vi "Initial Values-format and values-Live window.vi"() -> (13 "Values.Boolean":bool[](array[boolean]), 14 "Keys setup.DBL":T2=[{"key"="Control FPGA.Clock Freq (MHz)", "Save?"=TRUE, "Default"=240.0}, {"key"="DAQ FPGA.Clock Freq (MHz)", "Save?"=TRUE, "Default"=240.0}], 15 "Values.DBL":dbl[](array[numeric]), 16 "Keys setup.String":T3=[{"key"="Control FPGA.MAC address", "Save?"=TRUE, "Default"="AABBCCDDEEFF"}, {"key"="DAQ FPGA.Target", "Save?"=TRUE, "Default"="RIO0"}, {"key"="XY Stage.COM port", "Save?"=TRUE, "Default"="COM7"}, {"key"="DAQmx Chan.Pockels Control", "Save?"=TRUE, "Default"=""}, {"key"="DAQmx Chan.Hard Shutter", "Save?"=TRUE, "Default"=""}, {"key"="DAQmx Chan.PMT 1", "Save?"=TRUE, "Default"=""}, {"key"="DAQmx Chan.PMT 2", "Save?"=TRUE, "Default"=""}, {"key"="DAQmx Chan.Encoder Trigger", "Save?"=TRUE, "Default"=""}, {"key"="DAQmx Chan.Optional Trigger 1", "Save?"=TRUE, "Default"=""}, {"key"="DAQmx Chan.Optional Trigger 2", "Save?"=TRUE, "Default"=""}, {"key"="DAQmx Chan.Optional Trigger 3", "Save?"=TRUE, "Default"=""}], 17 "Values.Strings":string[](array[string]), 18 "Keys setup.Boolean":T1, 19 "error out":errorcluster)   [LabVIEW 2017]
uses:
  Typedefs/Ini file interface (String).ctl
  Typedefs/Ini file interface (DBL).ctl
  Typedefs/Ini file interface (Boolean).ctl
  User Interface/Globals/gl_Windows Ctrl refs.vi
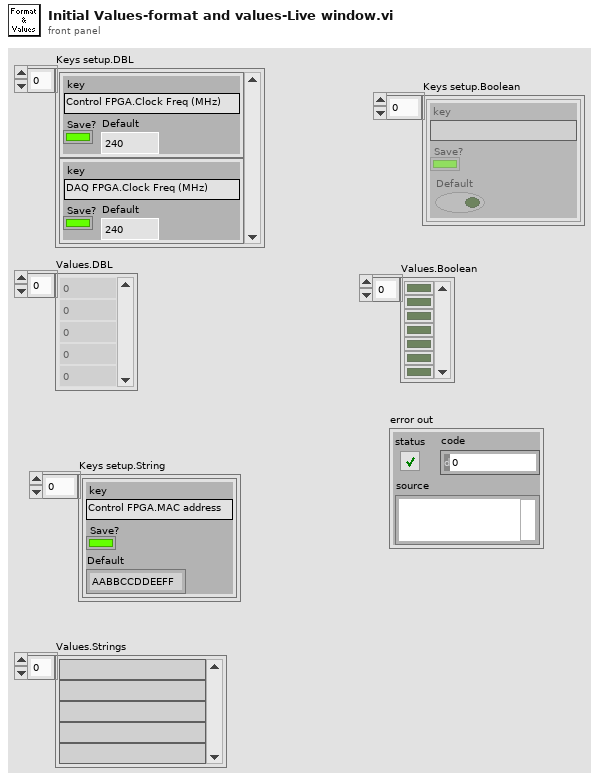
[diagram p1: front panel]
types:
  T1 = typedef "Ini file interface (Boolean).ctl" = cluster{"key":string, "Save?":bool, "Default":bool}[]
  T2 = typedef "Ini file interface (DBL).ctl" = cluster{"key":string, "Save?":bool, "Default":dbl}[]
  T3 = typedef "Ini file interface (String).ctl" = cluster{"key":string, "Save?":bool, "Default":string}[]
  T4 = typedef "Live window-ctrl refs.ctl" = cluster{"This VI":refnum<vi>, "Pane":refnum<vi>, "Show REF Image Left":refnum<vi>, "Show REF Image Right":refnum<vi>, "Snapshot":refnum<vi>, "Left Image Palette":refnum<vi>, "Right Image Palette":refnum<vi>, "Left Channel":refnum<vi>, "Right Channel":refnum<vi>, "Left image intensity":refnum<vi>, "Right image intensity":refnum<vi>, "Left Image Display":T5, "Right Image Display":T5, "Refresh rate ind (Hz)":refnum<vi>, "Acq rate ind (Hz)":refnum<vi>, "Stop (ind)":refnum<vi>}
  T5 = typedef "Image display ref.ctl" = refnum<vi>
  T6 = typedef "Channel Selector.ctl" = enum16{"Red Channel", "Green Channel", "Blended"}
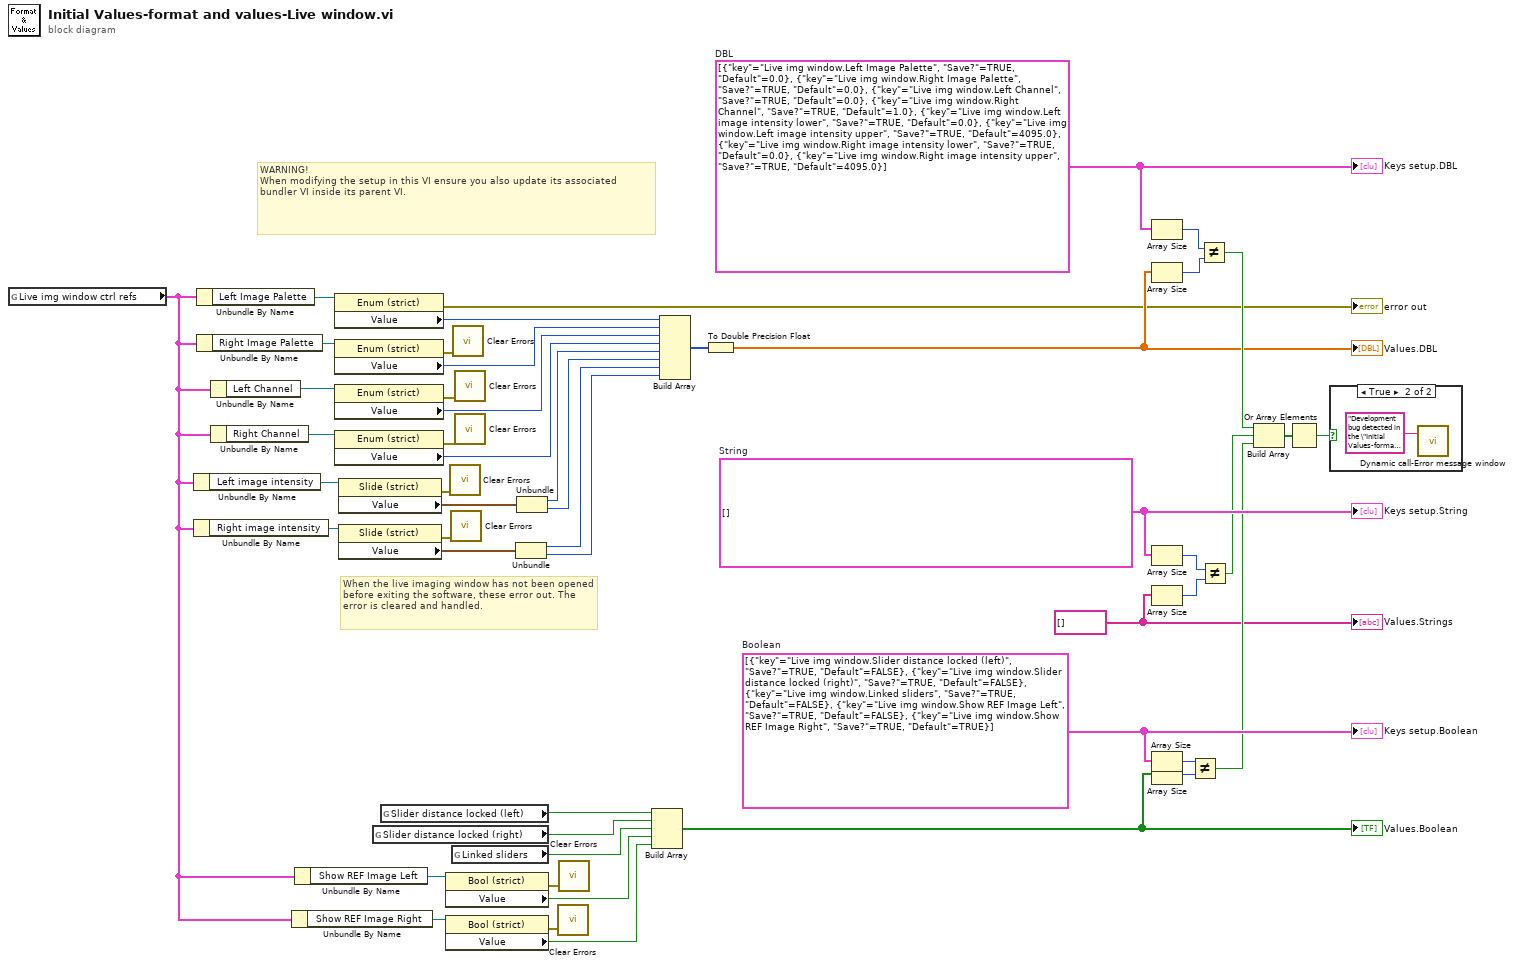
[diagram p0: block diagram]
diagram:
  w34 = string[] [] ("appended array")
  w47 = T1 [{"key"="Live img window.Slider distance locked (left)", "Save?"=TRUE, "Default"=FALSE}, {"key"="Live img window.Slider distance locked (right)", "Save?"=TRUE, "Default"=FALSE}, {"key"="Live img window.Linked sliders", "Save?"=TRUE, "Default"=FALSE}, {"key"="Live img window.Show REF Image Left", "Save?"=TRUE, "Default"=FALSE}, {"key"="Live img window.Show REF Image Right", "Save?"=TRUE, "Default"=TRUE}]  # Boolean
  w50 = T3 []  # String
  w49 = T2 [{"key"="Live img window.Left Image Palette", "Save?"=TRUE, "Default"=0.0}, {"key"="Live img window.Right Image Palette", "Save?"=TRUE, "Default"=0.0}, {"key"="Live img window.Left Channel", "Save?"=TRUE, "Default"=0.0}, {"key"="Live img window.Right Channel", "Save?"=TRUE, "Default"=1.0}, {"key"="Live img window.Left image intensity lower", "Save?"=TRUE, "Default"=0.0}, {"key"="Live img window.Left image intensity upper", "Save?"=TRUE, "Default"=4095.0}, {"key"="Live img window.Right image intensity lower", "Save?"=TRUE, "Default"=0.0}, {"key"="Live img window.Right image intensity upper", "Save?"=TRUE, "Default"=4095.0}]  # DBL
  # "When the live imaging window has not been opened before exiting the software, these error out. The error is cleared and handled."
  # "WARNING!\nWhen modifying the setup in this VI ensure you also update its associated bundler VI inside its parent VI."
  n1 = global read "gl_Windows Ctrl refs.vi" "Live img window ctrl refs"() -> (w5:T4)
  n2 = Unbundle By Name(w5) -> ("Left image intensity"=w24:refnum<vi>)
  n3 = Unbundle By Name(w5) -> ("Right image intensity"=w25:refnum<vi>)
  n4 = Unbundle By Name(w5) -> ("Left Image Palette"=w35:refnum<vi>)
  n5 = Unbundle By Name(w5) -> ("Right Image Palette"=w32:refnum<vi>)
  n6 = Unbundle By Name(w5) -> ("Left Channel"=w29:refnum<vi>)
  n7 = Unbundle By Name(w5) -> ("Right Channel"=w30:refnum<vi>)
  n8 = Unbundle By Name(w5) -> ("Show REF Image Right"=w6:refnum<vi>)
  n9 = Unbundle By Name(w5) -> ("Show REF Image Left"=w7:refnum<vi>)
  n10 = property class="Enum (strict)"(reference=w35) -> (error out=→"error out":errorcluster, "Value"=w33:enum16{"Gray", "Red", "Green"})  [unwired: 1 in, 1 out]
  n11 = property class="Enum (strict)"(reference=w32) -> (error out=w17:errorcluster, "Value"=w31:enum16{"Gray", "Red", "Green"})  [unwired: 1 in, 1 out]
  n12 = property class="Enum (strict)"(reference=w29) -> (error out=w16:errorcluster, "Value"=w28:T6)  [unwired: 1 in, 1 out]
  n13 = property class="Enum (strict)"(reference=w30) -> (error out=w15:errorcluster, "Value"=w27:T6)  [unwired: 1 in, 1 out]
  n14 = property class="Slide (strict)"(reference=w24) -> (error out=w14:errorcluster, "Value"=w23:cluster{i16, i16})  [unwired: 1 in, 1 out]
  n15 = property class="Slide (strict)"(reference=w25) -> (error out=w13:errorcluster, "Value"=w22:cluster{i16, i16})  [unwired: 1 in, 1 out]
  n16 = global read "gl_Windows Ctrl refs.vi" "Slider distance locked (right)"() -> (w10:bool)
  n17 = global read "gl_Windows Ctrl refs.vi" "Slider distance locked (left)"() -> (w11:bool)
  n18 = property class="Bool (strict)"(reference=w7) -> (error out=w2:errorcluster, "Value"=w4:bool)  [unwired: 1 in, 1 out]
  n19 = property class="Bool (strict)"(reference=w6) -> (error out=w1:errorcluster, "Value"=w3:bool)  [unwired: 1 in, 1 out]
  n20 = call <vilib>:"Clear Errors.vi"("error in (no error)"=w14) -> ()  [unwired: 5 in, 2 out]
  n21 = call <vilib>:"Clear Errors.vi"("error in (no error)"=w13) -> ()  [unwired: 5 in, 2 out]
  n22 = global read "gl_Windows Ctrl refs.vi" "Linked sliders"() -> (w8:bool)
  n23 = call <vilib>:"Clear Errors.vi"("error in (no error)"=w17) -> ()  [unwired: 5 in, 2 out]
  n24 = call <vilib>:"Clear Errors.vi"("error in (no error)"=w16) -> ()  [unwired: 5 in, 2 out]
  n25 = call <vilib>:"Clear Errors.vi"("error in (no error)"=w15) -> ()  [unwired: 5 in, 2 out]
  n26 = Unbundle(w22) -> (w19:i16, w18:i16)
  n27 = Unbundle(w23) -> (w21:i16, w20:i16)
  n28 = call <vilib>:"Clear Errors.vi"("error in (no error)"=w1) -> ()  [unwired: 5 in, 2 out]
  n29 = call <vilib>:"Clear Errors.vi"("error in (no error)"=w2) -> ()  [unwired: 5 in, 2 out]
  n30 = Build Array(w11, w10, w8, w4, w3) -> (w9:bool[])
  "Values.Boolean" <- w9
  n31 = Build Array(w33, w31, w28, w27, w21, w20, w19, w18) -> (w48:u16[])
  n32 = To Double Precision Float(number=w48) -> (double precision float=w26:dbl[])
  "Values.DBL" <- w26
  n33 = Array Size(array=w49) -> (size(s)=w44:i32)
  n34 = Array Size(array=w26) -> (size(s)=w43:i32)
  n35 = Array Size(array=w50) -> (size(s)=w46:i32)
  n36 = Array Size(array=w34) -> (size(s)=w45:i32)
  n37 = Array Size(array=w47) -> (size(s)=w42:i32)
  n38 = Array Size(array=w9) -> (size(s)=w41:i32)
  n39 = Not Equal?(x=w42, y=w41) -> (x != y?=w39:bool)
  n40 = Not Equal?(x=w44, y=w43) -> (x != y?=w37:bool)
  n41 = Not Equal?(x=w46, y=w45) -> (x != y?=w36:bool)
  n42 = Build Array(w37, w36, w39) -> (w40:bool[])
  n43 = Or Array Elements(Boolean array=w40) -> (logical OR=w38:bool)
  n44 = case shown="True" w38 {
    frame False {
    }
    frame True {
      n45 = call "Dynamic call-Error message window.vi"("Error Message"="Development bug detected in the \"Initial Values-format and values-Live window.vi\".\nPlease correct the set up in this VI.") -> ()  [unwired: 10 in, 1 out]
    }
  }
  "Keys setup.String" <- w50
  "Keys setup.DBL" <- w49
  "Values.Strings" <- w34
  "Keys setup.Boolean" <- w47
